vi "get sample rate.vi"(8 "error in (no error)":errorcluster, 11 "DeviceRefnum":u64) -> (0 "error out":errorcluster, 2 "Sample Rate (Hz)":u32, 3 "DeviceRefnum Out":u64)   [LabVIEW 2015, in "rtlsdr.lvlib"]
doc: "Get actual sample rate the device is configured to."
uses:
  rtlsdr.lvlib
  rtlsdr/rtlsdr.dll
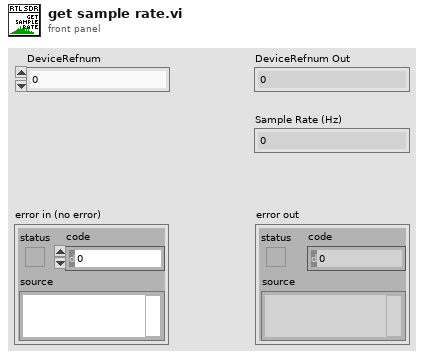
[diagram p1: front panel]
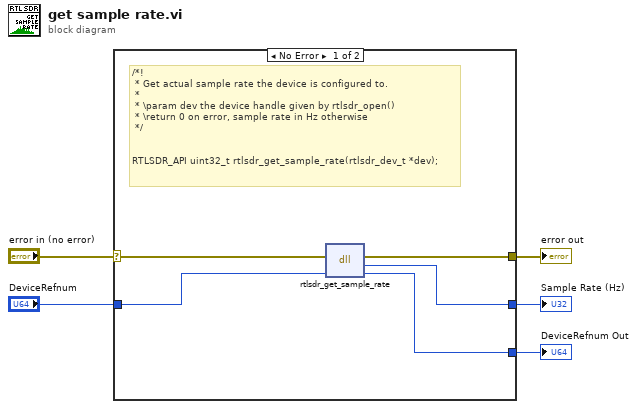
[diagram p0: block diagram]
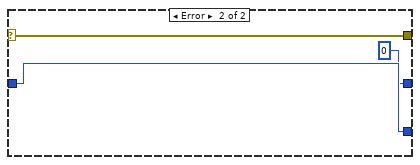
[diagram p2: hidden frame]
diagram:
  n1 = case shown="No Error" "error in (no error)" {
    selector: "error in (no error)" -> [w6 w13]
    tunnel: [w10 u32 0 ("return type")] -> w5
    tunnel: [w9 w13] -> w4
    tunnel: "DeviceRefnum" -> [w8 w12]
    tunnel: [w7 w12] -> w2
    frame No Error {
      # "/*!\n * Get actual sample rate the device is configured to.\n *\n * \\param dev the device handle given by rtlsdr_open()\n * \\return 0 on error, sample rate in Hz otherwise\n */\n\n\nRTLSDR_API uint32_t rtlsdr_get_sample_rate(rtlsdr_dev_t *dev);"
      n2 = dll-call lib="C:/Users/TheDoctor/Documents/Projects/Labview Libraries/rtlsdr/rtlsdr.*" fn="rtlsdr_get_sample_rate"(error in=w6, "DeviceRefnum"=w8) -> (error out=w9:errorcluster, "return type"=w10:u32, "DeviceRefnum"=w7:u64)  [unwired: 2 in, 1 out]
    }
    frame Error {
    }
  }
  "Sample Rate (Hz)" <- w5
  "error out" <- w4
  "DeviceRefnum Out" <- w2
